vi "Interseccion de Semaforos.vi"() -> ()   [LabVIEW 2020]
panel:
  out "Tiempo Transcurrido\n(milisegundos)":dbl
  in  "Detener \nPrograma":bool
  in  "Escoja el Tiempo":dbl(slide) scale=0.0..1.0
  out "V2":bool
  out "A2":bool
  out "R2":bool
  out "V1":bool
  out "A1":bool
  out "R1":bool
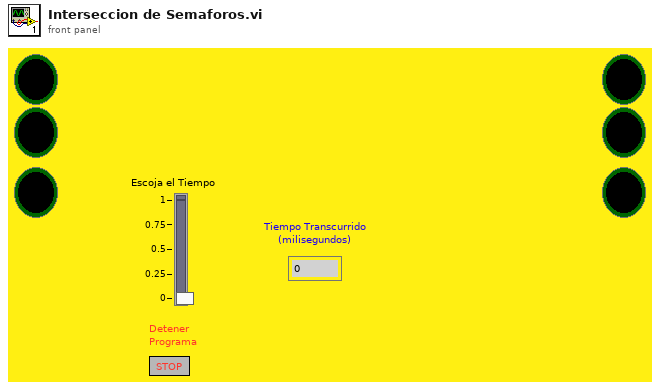
[diagram p1: front panel]
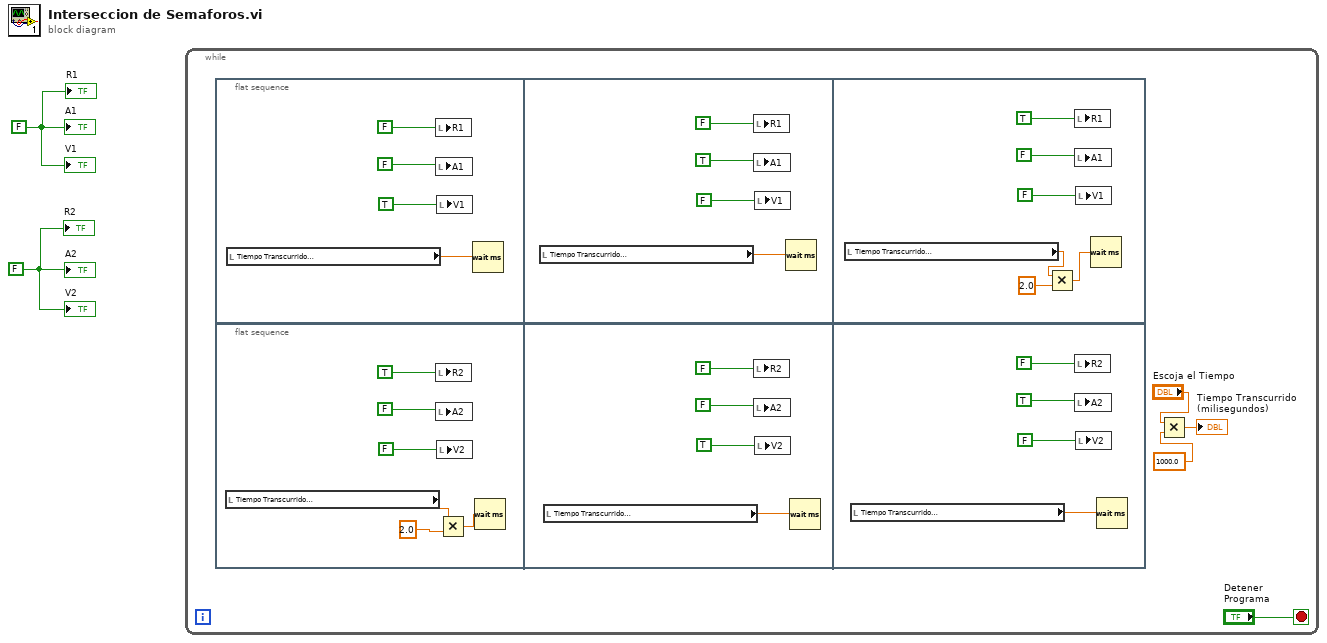
[diagram p0: block diagram]
diagram:
  w1 = FALSE
  w2 = FALSE
  n1 = while {
    stop <- "Detener \nPrograma" stop-if-true
    n2 = flat-sequence {
      frame #0 {
        n3 = local read "Tiempo Transcurrido\n(milisegundos)"() -> (w21:dbl)
        n4 = local write "R1"(FALSE) -> ()
        n5 = local write "A1"(FALSE) -> ()
        n6 = local write "V1"(TRUE) -> ()
        n7 = Wait (ms)(milliseconds to wait=w21) -> ()  [unwired: 1 out]
      }
      frame #1 {
        n8 = local read "Tiempo Transcurrido\n(milisegundos)"() -> (w25:dbl)
        n9 = local write "R1"(FALSE) -> ()
        n10 = local write "A1"(TRUE) -> ()
        n11 = local write "V1"(FALSE) -> ()
        n12 = Wait (ms)(milliseconds to wait=w25) -> ()  [unwired: 1 out]
      }
      frame #2 {
        n13 = local read "Tiempo Transcurrido\n(milisegundos)"() -> (w29:dbl)
        n14 = Multiply(x=w29, y=2.0) -> (x*y=w31:dbl)
        n15 = local write "R1"(TRUE) -> ()
        n16 = local write "A1"(FALSE) -> ()
        n17 = local write "V1"(FALSE) -> ()
        n18 = Wait (ms)(milliseconds to wait=w31) -> ()  [unwired: 1 out]
      }
    }
    n19 = flat-sequence {
      frame #0 {
        n20 = local read "Tiempo Transcurrido\n(milisegundos)"() -> (w7:dbl)
        n21 = local write "R2"(TRUE) -> ()
        n22 = local write "A2"(FALSE) -> ()
        n23 = local write "V2"(FALSE) -> ()
        n24 = Multiply(x=w7, y=2.0) -> (x*y=w9:dbl)
        n25 = Wait (ms)(milliseconds to wait=w9) -> ()  [unwired: 1 out]
      }
      frame #1 {
        n26 = local read "Tiempo Transcurrido\n(milisegundos)"() -> (w13:dbl)
        n27 = local write "R2"(FALSE) -> ()
        n28 = local write "A2"(FALSE) -> ()
        n29 = local write "V2"(TRUE) -> ()
        n30 = Wait (ms)(milliseconds to wait=w13) -> ()  [unwired: 1 out]
      }
      frame #2 {
        n31 = local read "Tiempo Transcurrido\n(milisegundos)"() -> (w17:dbl)
        n32 = local write "R2"(FALSE) -> ()
        n33 = local write "A2"(TRUE) -> ()
        n34 = local write "V2"(FALSE) -> ()
        n35 = Wait (ms)(milliseconds to wait=w17) -> ()  [unwired: 1 out]
      }
    }
    n36 = Multiply(x="Escoja el Tiempo", y=1000.0) -> (x*y=→"Tiempo Transcurrido\n(milisegundos)":dbl)
  }
  "R1" <- w2
  "A1" <- w2
  "V1" <- w2
  "R2" <- w1
  "A2" <- w1
  "V2" <- w1
